vi "PC Main.vi"() -> ()   [LabVIEW 2017]
uses:
  <vilib>/Platform/TimedLoop/XDataNode/timing_clust.ctl
  <vilib>/Platform/TimedLoop/XDataNode/nitl_modes.ctl
  <vilib>/Platform/TimedLoop/XDataNode/wakeup.ctl
  <vilib>/Analysis/baseanly.llb/Mean (DBL).vi
  <vilib>/platform/TimedLoop/XDataNode/XDataNode.xnode
  <userlib>/dxl_x86_c/dxl_x86_c.lvlib
  <vilib>/Analysis/NI_AALBase.lvlib
  <vilib>/Platform/TimedLoop/XDataNode/XDNodeRunTimeDep.lvlib
panel:
  out "mu 2":dbl=159.53475918016642
  out "mu 1":dbl=131.25865463967781
  out "Foward Kinematics":cluster{dbl[], dbl[]}(graph)={[0.0, 0.0, 13.983329390294564, 18.201151856471842, -2.133372344390357, 0.0], [0.0, 4.5, -20.906032731666787, -49.59766868439368, -28.921423243682018, 0.0]}
  in  "w":dbl=4.5
  in  "b 1":dbl=29.0
  in  "a 1":dbl=29.0
  out "theta 2":dbl=151.171875
  out "theta 1":dbl=184.21875
  out "variable 2":dbl=-1.4545454545454533
  out "value : MX\npresent speed 2":u16
  out "value : MX\npresent position 2":u16=2744
  out "value : MX\ngoal torque 2":u16
  out "value: MX\npresent load 2":u16=56
  out "dynamixel_id 2":u8=11
  in  "ticks":i32=5
  in  "trigger":dbl=30.0
  out "variable 1":dbl=0.581818181818182
  out "value : MX\npresent speed 1":u16
  in  "torque":dbl=120.0
  out "CONTROL MODE":string="POSITION LOCK"
  out "value: MX\npresent load 1":u16=1032
  out "ADDR_MX_\nPRESENT_LOAD":u16=40
  out "ADDR_MX_\nPRESENT_SPEED":u16=38
  out "ADDR_MX_\nTORQUE_CONTROL_MODE_ENABLE":u16=70
  out "value : MX\ngoal torque 1":u16
  in  "terminate":bool
  out "value : MX\npresent position 1":u16=3120
  out "baud_rate":i32=57600
  out "dynamixel_id 1":u8=12
  out "protocol_version":dbl=1.0
  out "port_num":i32
  out "ADDR_MX_\nTORQUE_ENABLE":u16=24
  out "ADDR_MX_\nGOAL_TORQUE":u16=71
  out "ADDR_MX_\nPRESENT_POSITION":u16=36
  out "device_name":string="COM3"
  out "dynamixel_comm_result":string="[TxRxResult] Communication success."
  out "dynamixel_error":string
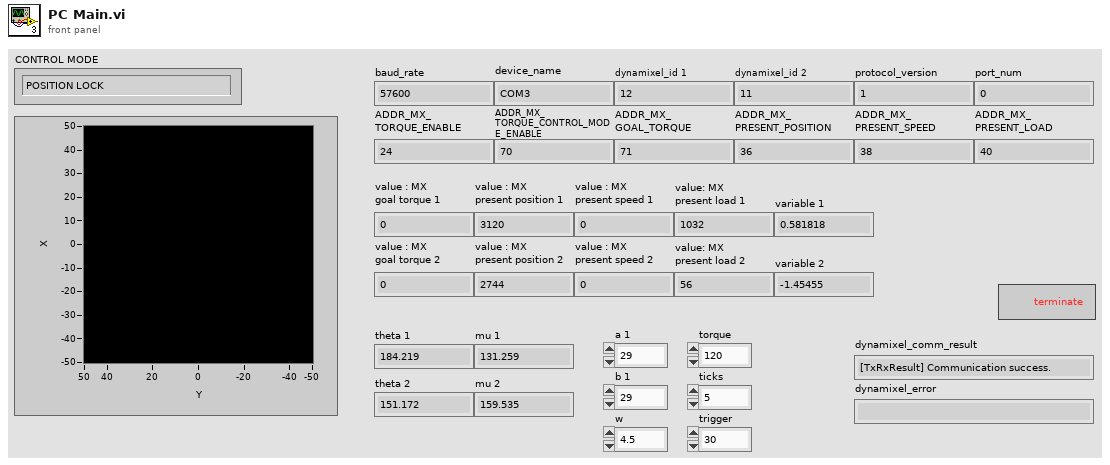
[diagram p1: front panel]
types:
  T1 = typedef "XDNodeRunTimeDep.lvlib/timing_clust.ctl" = cluster{"Expected End [f-1]":u64, "Actual End [f-1]":u64, "Finished Late? [f-1]":bool, "Expected End [i-1]":u64, "Actual End [i-1]":u64, "Finished Late? [i-1]":bool, "Expected Start [i]":u64, "Actual Start [i]":u64, "Expected Start [f]":u64, "Actual Start [f]":u64, "Source Name":string, "Structure Name":string, "Period":i64, "Deadline":i64, "Offset":i64, "Start":i64, "Priority":i32, "Timeout":i32, "Mode":T2, "Wakeup Reason":T3, "Error":errorcluster, "Source Type":string, "Secondary Source Type":string, "Global End Time":u64, "Global Start Time":u64, "Frame Duration":u64, "Iteration Duration":u64, "Assigned CPU":i32, "I/O Scan Engine Mode":u32}
  T2 = typedef "XDNodeRunTimeDep.lvlib/nitl_modes.ctl" = enum32{"No Change", "Process missed periods, maintain original phase", "Discard missed periods, maintain original phase", "Process missed periods, ignore original phase", "Discard missed periods, ignore original phase"}
  T3 = typedef "XDNodeRunTimeDep.lvlib/wakeup.ctl" = enum32{"Normal", "Aborted", "Asynchronous wakeup", "Timing source error", "Timed loop error", "Timeout"}
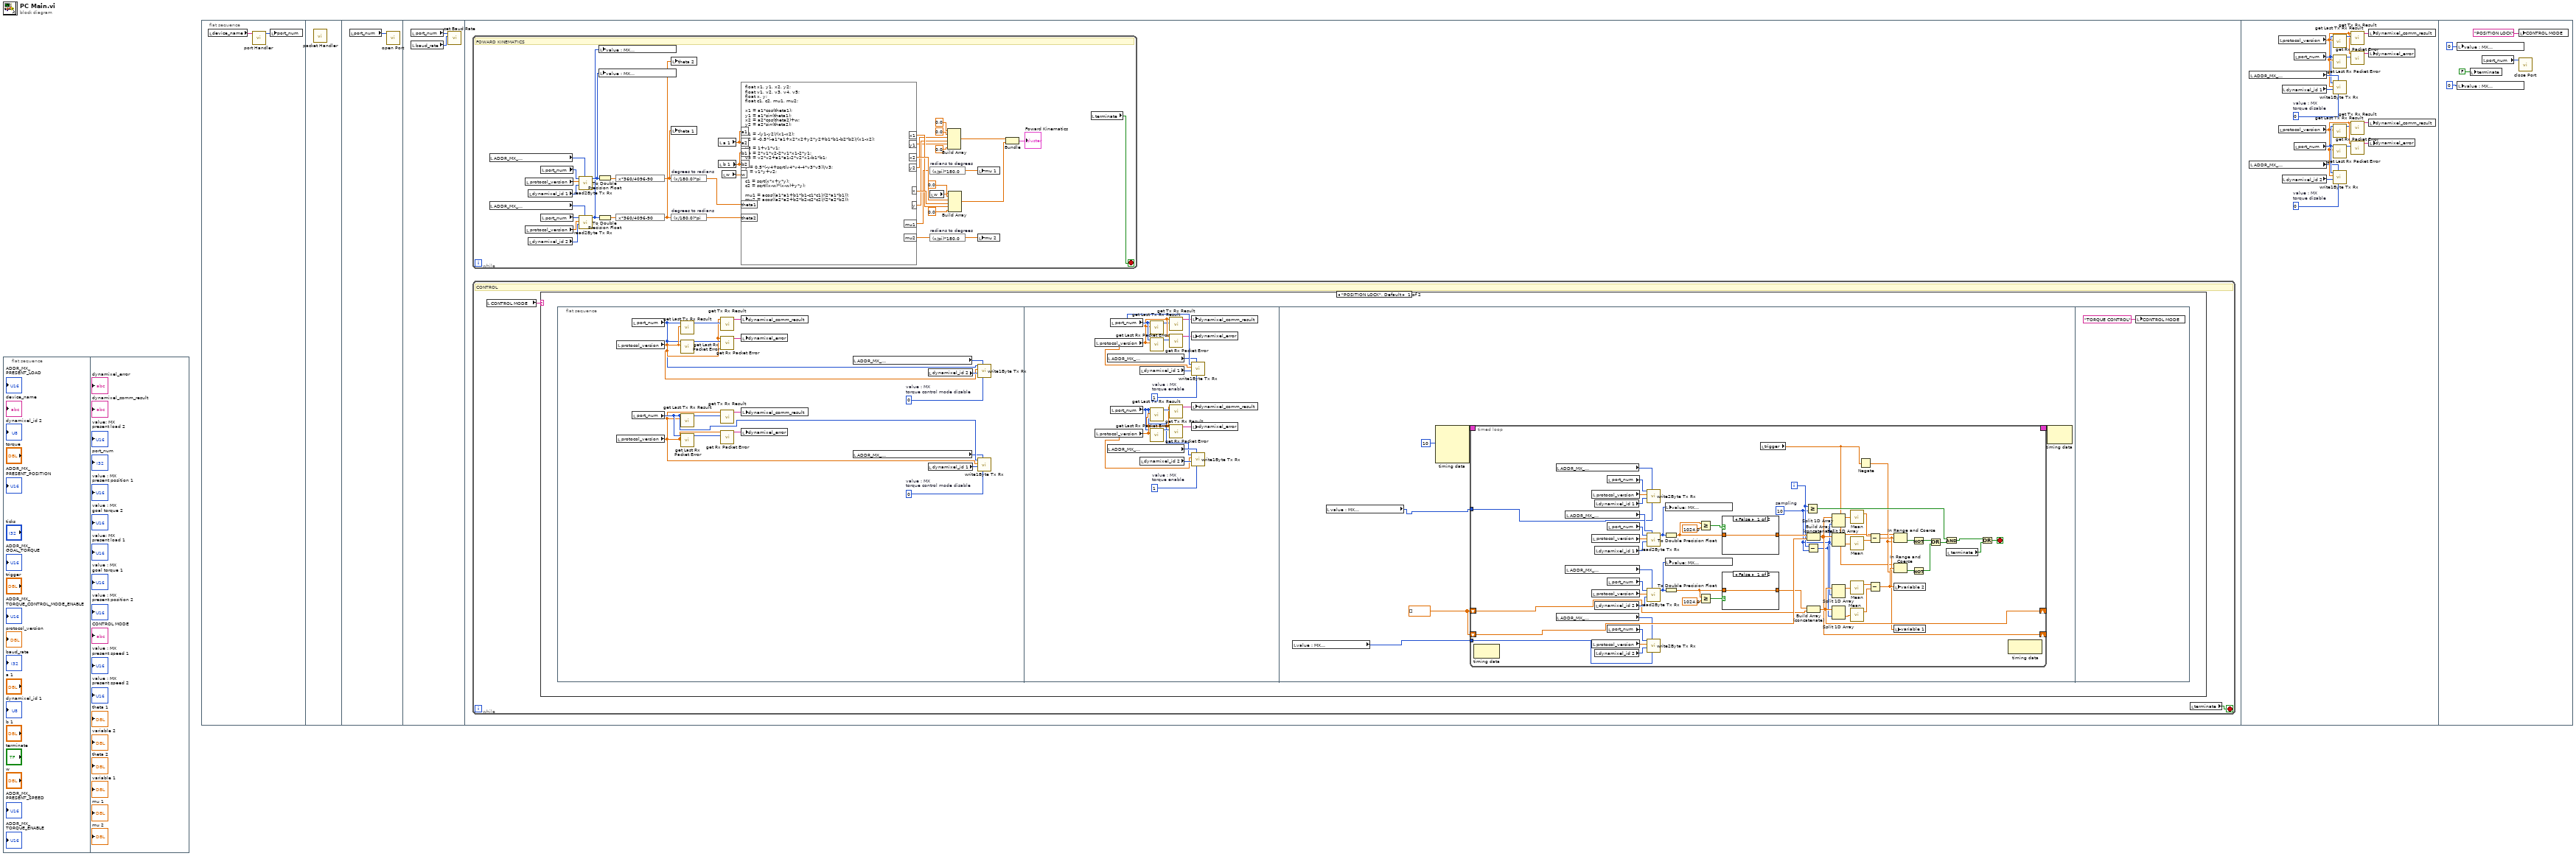
[diagram p0: block diagram]
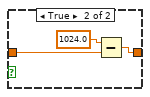
[diagram p2: hidden frame]
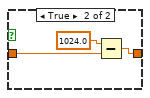
[diagram p3: hidden frame]
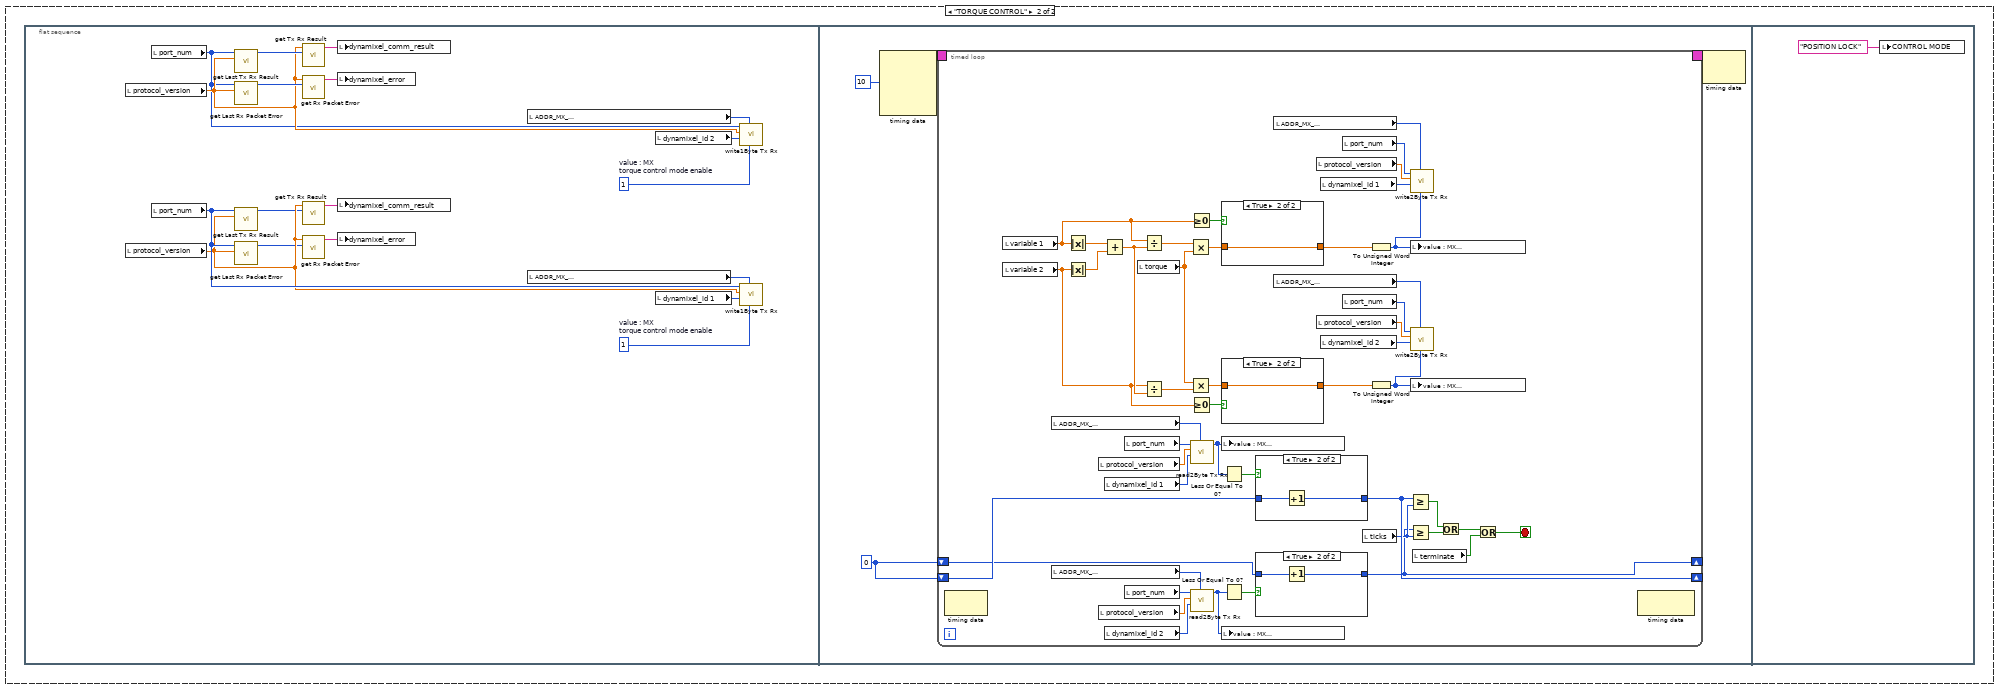
[diagram p4: hidden frame]
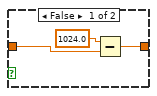
[diagram p5: hidden frame]
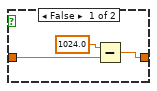
[diagram p6: hidden frame]
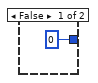
[diagram p7: hidden frame]
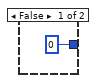
[diagram p8: hidden frame]
diagram:
  n1 = flat-sequence {
    frame #0 {
    }
    frame #1 {
    }
  }
  n2 = flat-sequence {
    frame #0 {
      n3 = local read "device_name"() -> (w2:string)
      n4 = call <userlib>:"port Handler.vi"("port_name"=w2) -> ("function return"=w1:i32)  [unwired: 10 in]
      n5 = local write "port_num"(w1) -> ()
    }
    frame #1 {
      n6 = call <userlib>:"packet Handler.vi"() -> ()  [unwired: 12 in]
    }
    frame #2 {
      n7 = local read "port_num"() -> (w3:i32)
      n8 = call <userlib>:"open Port.vi"("port_num"=w3) -> ()  [unwired: 10 in, 1 out]
    }
    frame #3 {
      n9 = local read "port_num"() -> (w4:i32)
      n10 = local read "baud_rate"() -> (w5:i32)
      n11 = call <userlib>:"set Baud Rate.vi"("baudrate"=w5, "port_num"=w4) -> ()  [unwired: 9 in, 1 out]
    }
    frame #4 {
      n12 = while {
        stop <- w6 stop-if-true
        # "FOWARD KINEMATICS"
        n13 = local read "ADDR_MX_\nPRESENT_POSITION"() -> (w44:u16)
        n14 = local read "ADDR_MX_\nPRESENT_POSITION"() -> (w37:u16)
        n15 = local read "protocol_version"() -> (w42:dbl)
        n16 = local read "protocol_version"() -> (w39:dbl)
        n17 = local read "dynamixel_id 1"() -> (w41:u8)
        n18 = local read "dynamixel_id 2"() -> (w40:u8)
        n19 = local read "port_num"() -> (w43:i32)
        n20 = local read "port_num"() -> (w38:i32)
        n21 = call <userlib>:"read2Byte Tx Rx.vi"("address"=w44, "id"=w41, "protocol_version"=w42, "port_num"=w43) -> ("function return"=w36:u16)  [unwired: 7 in]
        n22 = call <userlib>:"read2Byte Tx Rx.vi"("address"=w37, "id"=w40, "protocol_version"=w39, "port_num"=w38) -> ("function return"=w34:u16)  [unwired: 7 in]
        n23 = To Double Precision Float(number=w36) -> (double precision float=w35:dbl)
        n24 = To Double Precision Float(number=w34) -> (double precision float=w33:dbl)
        n25 = local write "value : MX\npresent position 2"(w34) -> ()
        n26 = local write "value : MX\npresent position 1"(w36) -> ()
        n27 = expression code="x*360/4096-90"(w35) -> (w17:dbl)
        n28 = expression code="x*360/4096-90"(w33) -> (w19:dbl)
        n29 = local write "theta 2"(w19) -> ()
        n30 = local write "theta 1"(w17) -> ()
        n31 = expression code="(x/180.0)*pi" "degrees to radians"(w17) -> (w16:dbl)
        n32 = expression code="(x/180.0)*pi" "degrees to radians"(w19) -> (w18:dbl)
        n33 = local read "a 1"() -> (w32:dbl)
        n34 = local read "b 1"() -> (w30:dbl)
        n35 = local read "w"() -> (w31:dbl)
        n36 = formula code="float x1, y1, x2, y2;\nfloat v1, v2, v3, v4, v5;\nfloat x, y;\nfloat c1, c2, mu1, mu2;\n\nx1 = a1*cos(theta1);\ny1 = a1*sin(theta1);\nx2 = a2*cos(theta2)+w;\ny2 = a2*sin(theta2);\n\nv1 = -(y1-y2)/(x1-x2);\nv2 = -0.5*(-a1*a1+x2*x2+y2*y2+b1*b1-b2*b2)/(x1-x2);\n\nv3 = 1+v1*v1;\nv4 = 2*v1*v2-2*v1*x1-2*y1;\nv5 = v2*v2+a1*a1-2*v2*x1-b1*b1;\n\ny = 0.5*(-v4+sqrt(v4*v4-4*v3*v5))/v3;\nx = v1*y+v2;\n\nc1 = sqrt(x*x+y*y);\nc2 = sqrt((x-w)*(x-w)+y*y);\n\nmu1 = acos((a1*a1+b1*b1-c1*c1)/(2*a1*b1));\nmu2 = acos((a2*a2+b2*b2-c2*c2)/(2*a2*b2));"("a1"=w32, "a2"=w32, "b1"=w30, "b2"=w30, "w"=w31, "theta1"=w16, "theta2"=w18) -> ("x1"=w26:dbl, "y1"=w23:dbl, "x2"=w28:dbl, "y2"=w25:dbl, "x"=w27:dbl, "y"=w24:dbl, "mu1"=w15:dbl, "mu2"=w14:dbl)
        n37 = expression code="(x/pi)*180.0" "radians to degrees"(w15) -> (w13:dbl)
        n38 = local read "w"() -> (w29:dbl)
        n39 = expression code="(x/pi)*180.0" "radians to degrees"(w14) -> (w12:dbl)
        n40 = Build Array(0.0 ("element"), 0.0 ("element"), w25, w24, w23, 0.0 ("element")) -> (w20:dbl[])
        n41 = Build Array(0.0 ("element"), w29, w28, w27, w26, 0.0 ("element")) -> (w21:dbl[])
        n42 = local write "mu 1"(w13) -> ()
        n43 = local write "mu 2"(w12) -> ()
        n44 = Bundle(w20, w21) -> (→"Foward Kinematics":cluster{dbl[], dbl[]})  [unwired: 1 in]
        n45 = local read "terminate"() -> (w6:bool)
      }
      n46 = while {
        stop <- w46 stop-if-true
        # "CONTROL"
        n47 = local read "CONTROL MODE"() -> (w45:string)
        n48 = case shown="\"POSITION LOCK\", Default" w45 {
          frame "POSITION LOCK", Default {
            n49 = flat-sequence {
              frame #0 {
                w47 = 0  # value : MX torque control mode disable
                w64 = 0  # value : MX torque control mode disable
                n50 = local read "protocol_version"() -> (w49:dbl)
                n51 = local read "protocol_version"() -> (w62:dbl)
                n52 = local read "port_num"() -> (w48:i32)
                n53 = local read "port_num"() -> (w63:i32)
                n54 = call <userlib>:"get Last Tx Rx Result.vi"("protocol_version"=w49, "port_num"=w48) -> ("function return"=w50:i32)  [unwired: 9 in]
                n55 = call <userlib>:"get Last Rx Packet Error.vi"("protocol_version"=w49, "port_num"=w48) -> ("function return"=w51:u8)  [unwired: 9 in]
                n56 = call <userlib>:"get Last Tx Rx Result.vi"("protocol_version"=w62, "port_num"=w63) -> ("function return"=w61:i32)  [unwired: 9 in]
                n57 = call <userlib>:"get Last Rx Packet Error.vi"("protocol_version"=w62, "port_num"=w63) -> ("function return"=w60:u8)  [unwired: 9 in]
                n58 = call <userlib>:"get Tx Rx Result.vi"("result"=w50, "protocol_version"=w49) -> ("function return"=w52:string)  [unwired: 9 in]
                n59 = call <userlib>:"get Rx Packet Error.vi"("error"=w51, "protocol_version"=w49) -> ("function return"=w53:string)  [unwired: 9 in]
                n60 = call <userlib>:"get Tx Rx Result.vi"("result"=w61, "protocol_version"=w62) -> ("function return"=w59:string)  [unwired: 9 in]
                n61 = call <userlib>:"get Rx Packet Error.vi"("error"=w60, "protocol_version"=w62) -> ("function return"=w58:string)  [unwired: 9 in]
                n62 = local write "dynamixel_comm_result"(w52) -> ()
                n63 = local write "dynamixel_error"(w53) -> ()
                n64 = local write "dynamixel_comm_result"(w59) -> ()
                n65 = local write "dynamixel_error"(w58) -> ()
                n66 = local read "ADDR_MX_\nTORQUE_CONTROL_MODE_ENABLE"() -> (w55:u16)
                n67 = local read "ADDR_MX_\nTORQUE_CONTROL_MODE_ENABLE"() -> (w56:u16)
                n68 = local read "dynamixel_id 2"() -> (w54:u8)
                n69 = local read "dynamixel_id 1"() -> (w57:u8)
                n70 = call <userlib>:"write1Byte Tx Rx.vi"("data"=w47, "address"=w55, "id"=w54, "protocol_version"=w49, "port_num"=w48) -> ()  [unwired: 7 in]
                n71 = call <userlib>:"write1Byte Tx Rx.vi"("data"=w64, "address"=w56, "id"=w57, "protocol_version"=w62, "port_num"=w63) -> ()  [unwired: 7 in]
              }
              frame #1 {
                w65 = 1  # value : MX torque enable
                w82 = 1  # value : MX torque enable
                n72 = local read "protocol_version"() -> (w80:dbl)
                n73 = local read "protocol_version"() -> (w67:dbl)
                n74 = local read "ADDR_MX_\nTORQUE_ENABLE"() -> (w74:u16)
                n75 = local read "ADDR_MX_\nTORQUE_ENABLE"() -> (w73:u16)
                n76 = local read "port_num"() -> (w81:i32)
                n77 = local read "port_num"() -> (w66:i32)
                n78 = local read "dynamixel_id 1"() -> (w75:u8)
                n79 = local read "dynamixel_id 2"() -> (w72:u8)
                n80 = call <userlib>:"get Last Tx Rx Result.vi"("protocol_version"=w80, "port_num"=w81) -> ("function return"=w79:i32)  [unwired: 9 in]
                n81 = call <userlib>:"get Last Rx Packet Error.vi"("protocol_version"=w80, "port_num"=w81) -> ("function return"=w78:u8)  [unwired: 9 in]
                n82 = call <userlib>:"get Last Tx Rx Result.vi"("protocol_version"=w67, "port_num"=w66) -> ("function return"=w68:i32)  [unwired: 9 in]
                n83 = call <userlib>:"get Last Rx Packet Error.vi"("protocol_version"=w67, "port_num"=w66) -> ("function return"=w69:u8)  [unwired: 9 in]
                n84 = call <userlib>:"get Tx Rx Result.vi"("result"=w79, "protocol_version"=w80) -> ("function return"=w77:string)  [unwired: 9 in]
                n85 = call <userlib>:"get Rx Packet Error.vi"("error"=w78, "protocol_version"=w80) -> ("function return"=w76:string)  [unwired: 9 in]
                n86 = call <userlib>:"get Tx Rx Result.vi"("result"=w68, "protocol_version"=w67) -> ("function return"=w70:string)  [unwired: 9 in]
                n87 = call <userlib>:"get Rx Packet Error.vi"("error"=w69, "protocol_version"=w67) -> ("function return"=w71:string)  [unwired: 9 in]
                n88 = local write "dynamixel_comm_result"(w77) -> ()
                n89 = local write "dynamixel_error"(w76) -> ()
                n90 = call <userlib>:"write1Byte Tx Rx.vi"("data"=w82, "address"=w74, "id"=w75, "protocol_version"=w80, "port_num"=w81) -> ()  [unwired: 7 in]
                n91 = local write "dynamixel_comm_result"(w70) -> ()
                n92 = local write "dynamixel_error"(w71) -> ()
                n93 = call <userlib>:"write1Byte Tx Rx.vi"("data"=w65, "address"=w73, "id"=w72, "protocol_version"=w67, "port_num"=w66) -> ()  [unwired: 7 in]
              }
              frame #2 {
                w85 = dbl[] []
                n94 = local read "value : MX\npresent position 2"() -> (w84:u16)
                n95 = local read "value : MX\npresent position 1"() -> (w83:u16)
                n96 = node-c288(i64 10 ("Period")) -> (w88:T1)  [unwired: 3 in]
                n97 = timed-loop {
                  shift-right: [w110] -> _
                  shift-left: w85 -> [w136]
                  shift-right: [w115] -> _
                  shift-left: w85 -> [w121]
                  timing: w88 -> [_]
                  timing-out: [_] -> w87
                  tunnel: w83 -> [w93]
                  tunnel: w84 -> [w92]
                  i -> [w103]
                  stop <- w118 stop-if-true
                  w102 = 10  # sampling
                  n98 = node-c288() -> ()  [unwired: 1 in, 1 out]
                  n99 = local read "ADDR_MX_\nPRESENT_POSITION"() -> (w101:u16)
                  n100 = local read "ADDR_MX_\nPRESENT_POSITION"() -> (w94:u16)
                  n101 = local read "ADDR_MX_\nPRESENT_LOAD"() -> (w144:u16)
                  n102 = local read "ADDR_MX_\nPRESENT_LOAD"() -> (w122:u16)
                  n103 = local read "protocol_version"() -> (w99:dbl)
                  n104 = local read "protocol_version"() -> (w141:dbl)
                  n105 = local read "protocol_version"() -> (w125:dbl)
                  n106 = local read "protocol_version"() -> (w96:dbl)
                  n107 = local read "dynamixel_id 1"() -> (w100:u8)
                  n108 = local read "dynamixel_id 1"() -> (w142:u8)
                  n109 = local read "dynamixel_id 2"() -> (w124:u8)
                  n110 = local read "dynamixel_id 2"() -> (w95:u8)
                  n111 = local read "port_num"() -> (w98:i32)
                  n112 = local read "port_num"() -> (w143:i32)
                  n113 = local read "port_num"() -> (w123:i32)
                  n114 = local read "port_num"() -> (w97:i32)
                  n115 = call <userlib>:"write2Byte Tx Rx.vi"("data"=w93, "address"=w101, "id"=w100, "protocol_version"=w99, "port_num"=w98) -> ()  [unwired: 7 in]
                  n116 = call <userlib>:"read2Byte Tx Rx.vi"("address"=w144, "id"=w142, "protocol_version"=w141, "port_num"=w143) -> ("function return"=w137:u16)  [unwired: 7 in]
                  n117 = call <userlib>:"read2Byte Tx Rx.vi"("address"=w122, "id"=w124, "protocol_version"=w125, "port_num"=w123) -> ("function return"=w129:u16)  [unwired: 7 in]
                  n118 = call <userlib>:"write2Byte Tx Rx.vi"("data"=w92, "address"=w94, "id"=w95, "protocol_version"=w96, "port_num"=w97) -> ()  [unwired: 7 in]
                  n119 = To Double Precision Float(number=w137) -> (double precision float=w138:dbl)
                  n120 = To Double Precision Float(number=w129) -> (double precision float=w128:dbl)
                  n121 = local write "value: MX\npresent load 1"(w137) -> ()
                  n122 = local write "value: MX\npresent load 2"(w129) -> ()
                  n123 = Greater Or Equal?(x=w138, y=1024.0) -> (x >= y?=w139:bool)
                  n124 = Greater Or Equal?(x=w128, y=1024.0) -> (x >= y?=w127:bool)
                  n125 = case shown="False" w139 {
                    tunnel: w138 -> [w151 w153]
                    tunnel: [w151 w152] -> w134
                    frame False {
                    }
                    frame True {
                      n126 = Subtract(x=1024.0, y=w153) -> (x-y=w152:dbl)
                    }
                  }
                  n127 = case shown="False" w127 {
                    tunnel: w128 -> [w147 w149]
                    tunnel: [w147 w148] -> w131
                    frame False {
                    }
                    frame True {
                      n128 = Subtract(x=1024.0, y=w149) -> (x-y=w148:dbl)
                    }
                  }
                  n129 = local read "trigger"() -> (w89:dbl)
                  n130 = Greater Or Equal?(x=w103, y=w102) -> (x >= y?=w104:bool)
                  n131 = Subtract(x=w103, y=w102) -> (x-y=w109:i32)
                  n132 = Build Array (concatenate)(w134, w136) -> (w110:dbl[])
                  n133 = Build Array (concatenate)(w131, w121) -> (w115:dbl[])
                  n134 = Split 1D Array(array=w110, index=w102) -> (first subarray=w135:dbl[])  [unwired: 1 out]
                  n135 = Split 1D Array(array=w110, index=w109) -> (second subarray=w111:dbl[])  [unwired: 1 out]
                  n136 = Split 1D Array(array=w115, index=w102) -> (first subarray=w130:dbl[])  [unwired: 1 out]
                  n137 = Split 1D Array(array=w115, index=w109) -> (second subarray=w116:dbl[])  [unwired: 1 out]
                  n138 = call-poly <vilib>:"Mean.vi"("X"=w135) -> ("mean"=w108:dbl)  [unwired: 1 out]
                  n139 = call-poly <vilib>:"Mean.vi"("X"=w111) -> ("mean"=w107:dbl)  [unwired: 1 out]
                  n140 = call-poly <vilib>:"Mean.vi"("X"=w130) -> ("mean"=w114:dbl)  [unwired: 1 out]
                  n141 = call-poly <vilib>:"Mean.vi"("X"=w116) -> ("mean"=w113:dbl)  [unwired: 1 out]
                  n142 = Negate(x=w89) -> (-x=w90:dbl)
                  n143 = Subtract(x=w108, y=w107) -> (x-y=w106:dbl)
                  n144 = Subtract(x=w114, y=w113) -> (x-y=w112:dbl)
                  n145 = In Range and Coerce(upper limit=w89, x=w106, lower limit=w90) -> (In Range?=w133:bool)  [unwired: 1 out]
                  n146 = In Range and Coerce(upper limit=w89, x=w112, lower limit=w90) -> (In Range?=w132:bool)  [unwired: 1 out]
                  n147 = local write "variable 2"(w112) -> ()
                  n148 = local write "variable 1"(w106) -> ()
                  n149 = Not(x=w133) -> (.not. x?=w117:bool)
                  n150 = Not(x=w132) -> (.not. x?=w120:bool)
                  n151 = Or(x=w117, y=w120) -> (x .or. y?=w105:bool)
                  n152 = And(x=w104, y=w105) -> (x .and. y?=w91:bool)
                  n153 = local read "terminate"() -> (w119:bool)
                  n154 = Or(x=w91, y=w119) -> (x .or. y?=w118:bool)
                  n155 = node-c288() -> ()  [unwired: 1 in, 1 out]
                }
                n156 = node-c288(w87) -> ()  [unwired: 1 out]
              }
              frame #3 {
                n157 = local write "CONTROL MODE"("TORQUE CONTROL" ("mode")) -> ()
              }
            }
          }
          frame "TORQUE CONTROL" {
            n158 = flat-sequence {
              frame #0 {
                w168 = 1  # value : MX torque control mode enable
                w169 = 1  # value : MX torque control mode enable
                n159 = local read "protocol_version"() -> (w161:dbl)
                n160 = local read "protocol_version"() -> (w176:dbl)
                n161 = local read "port_num"() -> (w160:i32)
                n162 = local read "port_num"() -> (w177:i32)
                n163 = call <userlib>:"get Last Tx Rx Result.vi"("protocol_version"=w161, "port_num"=w160) -> ("function return"=w162:i32)  [unwired: 9 in]
                n164 = call <userlib>:"get Last Rx Packet Error.vi"("protocol_version"=w161, "port_num"=w160) -> ("function return"=w163:u8)  [unwired: 9 in]
                n165 = call <userlib>:"get Last Tx Rx Result.vi"("protocol_version"=w176, "port_num"=w177) -> ("function return"=w175:i32)  [unwired: 9 in]
                n166 = call <userlib>:"get Last Rx Packet Error.vi"("protocol_version"=w176, "port_num"=w177) -> ("function return"=w174:u8)  [unwired: 9 in]
                n167 = call <userlib>:"get Tx Rx Result.vi"("result"=w162, "protocol_version"=w161) -> ("function return"=w164:string)  [unwired: 9 in]
                n168 = call <userlib>:"get Rx Packet Error.vi"("error"=w163, "protocol_version"=w161) -> ("function return"=w165:string)  [unwired: 9 in]
                n169 = call <userlib>:"get Tx Rx Result.vi"("result"=w175, "protocol_version"=w176) -> ("function return"=w173:string)  [unwired: 9 in]
                n170 = call <userlib>:"get Rx Packet Error.vi"("error"=w174, "protocol_version"=w176) -> ("function return"=w172:string)  [unwired: 9 in]
                n171 = local write "dynamixel_comm_result"(w164) -> ()
                n172 = local write "dynamixel_error"(w165) -> ()
                n173 = local write "dynamixel_comm_result"(w173) -> ()
                n174 = local write "dynamixel_error"(w172) -> ()
                n175 = local read "ADDR_MX_\nTORQUE_CONTROL_MODE_ENABLE"() -> (w167:u16)
                n176 = local read "ADDR_MX_\nTORQUE_CONTROL_MODE_ENABLE"() -> (w170:u16)
                n177 = local read "dynamixel_id 2"() -> (w166:u8)
                n178 = local read "dynamixel_id 1"() -> (w171:u8)
                n179 = call <userlib>:"write1Byte Tx Rx.vi"("data"=w168, "address"=w167, "id"=w166, "protocol_version"=w161, "port_num"=w160) -> ()  [unwired: 7 in]
                n180 = call <userlib>:"write1Byte Tx Rx.vi"("data"=w169, "address"=w170, "id"=w171, "protocol_version"=w176, "port_num"=w177) -> ()  [unwired: 7 in]
              }
              frame #1 {
                w181 = 0
                n181 = node-c288(i64 10 ("Period")) -> (w180:T1)  [unwired: 3 in]
                n182 = timed-loop {
                  shift-right: [w218] -> _
                  shift-left: w181 -> [w219]
                  shift-right: [w207] -> _
                  shift-left: w181 -> [w211]
                  timing: w180 -> [_]
                  timing-out: [_] -> w179
                  stop <- w221 stop-if-true
                  n183 = node-c288() -> ()  [unwired: 1 in, 1 out]
                  n184 = local read "variable 1"() -> (w188:dbl)
                  n185 = local read "variable 2"() -> (w182:dbl)
                  n186 = local read "ADDR_MX_\nPRESENT_SPEED"() -> (w227:u16)
                  n187 = local read "ADDR_MX_\nPRESENT_SPEED"() -> (w212:u16)
                  n188 = Absolute Value(x=w188) -> (abs(x)=w190:dbl)
                  n189 = Absolute Value(x=w182) -> (abs(x)=w191:dbl)
                  n190 = local read "protocol_version"() -> (w224:dbl)
                  n191 = local read "protocol_version"() -> (w215:dbl)
                  n192 = Add(x=w190, y=w191) -> (x+y=w189:dbl)
                  n193 = local read "dynamixel_id 1"() -> (w225:u8)
                  n194 = local read "dynamixel_id 2"() -> (w214:u8)
                  n195 = local read "port_num"() -> (w226:i32)
                  n196 = local read "port_num"() -> (w213:i32)
                  n197 = local read "torque"() -> (w185:dbl)
                  n198 = Divide(x=w188, y=w189) -> (x/y=w187:dbl)
                  n199 = Divide(x=w182, y=w189) -> (x/y=w186:dbl)
                  n200 = Multiply(x=w187, y=w185) -> (x*y=w183:dbl)
                  n201 = Multiply(x=w185, y=w186) -> (x*y=w184:dbl)
                  n202 = Greater Or Equal To 0?(x=w188) -> (x >= 0?=w205:bool)
                  n203 = Greater Or Equal To 0?(x=w182) -> (x >= 0?=w192:bool)
                  n204 = call <userlib>:"read2Byte Tx Rx.vi"("address"=w227, "id"=w225, "protocol_version"=w224, "port_num"=w226) -> ("function return"=w223:u16)  [unwired: 7 in]
                  n205 = call <userlib>:"read2Byte Tx Rx.vi"("address"=w212, "id"=w214, "protocol_version"=w215, "port_num"=w213) -> ("function return"=w216:u16)  [unwired: 7 in]
                  n206 = case shown="True" w205 {
                    tunnel: [w232 w235] -> w200
                    tunnel: w183 -> [w234 w235]
                    frame False {
                      n207 = Subtract(x=1024.0, y=w234) -> (x-y=w232:dbl)
                    }
                    frame True {
                    }
                  }
                  n208 = case shown="True" w192 {
                    tunnel: [w228 w231] -> w197
                    tunnel: w184 -> [w230 w231]
                    frame False {
                      n209 = Subtract(x=1024.0, y=w230) -> (x-y=w228:dbl)
                    }
                    frame True {
                    }
                  }
                  n210 = local write "value : MX\npresent speed 1"(w223) -> ()
                  n211 = local write "value : MX\npresent speed 2"(w216) -> ()
                  n212 = Less Or Equal To 0?(x=w223) -> (x <= 0?=w220:bool)
                  n213 = Less Or Equal To 0?(x=w216) -> (x <= 0?=w217:bool)
                  n214 = case shown="True" w220 {
                    tunnel: w219 -> [_ w243]
                    tunnel: [0 w242] -> w218
                    frame False {
                    }
                    frame True {
                      n215 = Increment(x=w243) -> (x+1=w242:i32)
                    }
                  }
                  n216 = case shown="True" w217 {
                    tunnel: w211 -> [_ w240]
                    tunnel: [0 w239] -> w207
                    frame False {
                    }
                    frame True {
                      n217 = Increment(x=w240) -> (x+1=w239:i32)
                    }
                  }
                  n218 = local read "ADDR_MX_\nGOAL_TORQUE"() -> (w201:u16)
                  n219 = local read "ADDR_MX_\nGOAL_TORQUE"() -> (w196:u16)
                  n220 = local read "protocol_version"() -> (w203:dbl)
                  n221 = local read "protocol_version"() -> (w194:dbl)
                  n222 = local read "dynamixel_id 1"() -> (w202:u8)
                  n223 = local read "dynamixel_id 2"() -> (w195:u8)
                  n224 = local read "port_num"() -> (w204:i32)
                  n225 = local read "port_num"() -> (w193:i32)
                  n226 = local read "ticks"() -> (w210:i32)
                  n227 = To Unsigned Word Integer(number=w200) -> (unsigned 16bit integer=w199:u16)
                  n228 = To Unsigned Word Integer(number=w197) -> (unsigned 16bit integer=w198:u16)
                  n229 = Greater Or Equal?(x=w218, y=w210) -> (x >= y?=w209:bool)
                  n230 = Greater Or Equal?(x=w207, y=w210) -> (x >= y?=w208:bool)
                  n231 = call <userlib>:"write2Byte Tx Rx.vi"("data"=w199, "address"=w201, "id"=w202, "protocol_version"=w203, "port_num"=w204) -> ()  [unwired: 7 in]
                  n232 = local write "value : MX\ngoal torque 1"(w199) -> ()
                  n233 = call <userlib>:"write2Byte Tx Rx.vi"("data"=w198, "address"=w196, "id"=w195, "protocol_version"=w194, "port_num"=w193) -> ()  [unwired: 7 in]
                  n234 = local write "value : MX\ngoal torque 2"(w198) -> ()
                  n235 = local read "terminate"() -> (w222:bool)
                  n236 = Or(x=w209, y=w208) -> (x .or. y?=w206:bool)
                  n237 = Or(x=w206, y=w222) -> (x .or. y?=w221:bool)
                  n238 = node-c288() -> ()  [unwired: 1 in, 1 out]
                }
                n239 = node-c288(w179) -> ()  [unwired: 1 out]
              }
              frame #2 {
                n240 = local write "CONTROL MODE"("POSITION LOCK" ("mode")) -> ()
              }
            }
          }
        }
        n241 = local read "terminate"() -> (w46:bool)
      }
    }
    frame #5 {
      w250 = 0  # value : MX torque disable
      w265 = 0  # value : MX torque disable
      n242 = local read "ADDR_MX_\nTORQUE_ENABLE"() -> (w266:u16)
      n243 = local read "ADDR_MX_\nTORQUE_ENABLE"() -> (w249:u16)
      n244 = local read "protocol_version"() -> (w259:dbl)
      n245 = local read "protocol_version"() -> (w256:dbl)
      n246 = local read "dynamixel_id 1"() -> (w264:u8)
      n247 = local read "dynamixel_id 2"() -> (w251:u8)
      n248 = local read "port_num"() -> (w258:i32)
      n249 = local read "port_num"() -> (w257:i32)
      n250 = call <userlib>:"get Last Tx Rx Result.vi"("protocol_version"=w259, "port_num"=w258) -> ("function return"=w260:i32)  [unwired: 9 in]
      n251 = call <userlib>:"get Last Rx Packet Error.vi"("protocol_version"=w259, "port_num"=w258) -> ("function return"=w261:u8)  [unwired: 9 in]
      n252 = call <userlib>:"write1Byte Tx Rx.vi"("data"=w265, "address"=w266, "id"=w264, "protocol_version"=w259, "port_num"=w258) -> ()  [unwired: 7 in]
      n253 = call <userlib>:"get Last Tx Rx Result.vi"("protocol_version"=w256, "port_num"=w257) -> ("function return"=w255:i32)  [unwired: 9 in]
      n254 = call <userlib>:"get Last Rx Packet Error.vi"("protocol_version"=w256, "port_num"=w257) -> ("function return"=w254:u8)  [unwired: 9 in]
      n255 = call <userlib>:"write1Byte Tx Rx.vi"("data"=w250, "address"=w249, "id"=w251, "protocol_version"=w256, "port_num"=w257) -> ()  [unwired: 7 in]
      n256 = call <userlib>:"get Tx Rx Result.vi"("result"=w260, "protocol_version"=w259) -> ("function return"=w262:string)  [unwired: 9 in]
      n257 = call <userlib>:"get Rx Packet Error.vi"("error"=w261, "protocol_version"=w259) -> ("function return"=w263:string)  [unwired: 9 in]
      n258 = call <userlib>:"get Tx Rx Result.vi"("result"=w255, "protocol_version"=w256) -> ("function return"=w253:string)  [unwired: 9 in]
      n259 = call <userlib>:"get Rx Packet Error.vi"("error"=w254, "protocol_version"=w256) -> ("function return"=w252:string)  [unwired: 9 in]
      n260 = local write "dynamixel_comm_result"(w262) -> ()
      n261 = local write "dynamixel_error"(w263) -> ()
      n262 = local write "dynamixel_comm_result"(w253) -> ()
      n263 = local write "dynamixel_error"(w252) -> ()
    }
    frame #6 {
      n264 = local write "value : MX\ngoal torque 2"(u16 0 ("value : MX (dial)\ngoal torque")) -> ()
      n265 = local write "value : MX\ngoal torque 1"(u16 0 ("value : MX (dial)\ngoal torque")) -> ()
      n266 = local write "terminate"(FALSE ("terminate")) -> ()
      n267 = local read "port_num"() -> (w271:i32)
      n268 = local write "CONTROL MODE"("POSITION LOCK" ("mode")) -> ()
      n269 = call <userlib>:"close Port.vi"("port_num"=w271) -> ()  [unwired: 11 in]
    }
  }
